vi "Get Pattern Data.vi"(9 "File Name":i32[](array[numeric]), 10 "Folder Name":string, 11 "Dispense.lvclass":refnum<class "Dispense.lvclass">) -> (3 "Dispense Out":refnum<class "Dispense.lvclass">)   [LabVIEW 2016, in "Dispense.lvclass"]
uses:
  Dispense.lvclass
  Dispense.lvclass/Dispense.ctl
panel:
  out "Timing Data (Go Down and Dispense)":T1(array[cluster])
  out "array":dbl[][](array[numeric])
  out "appended path":path
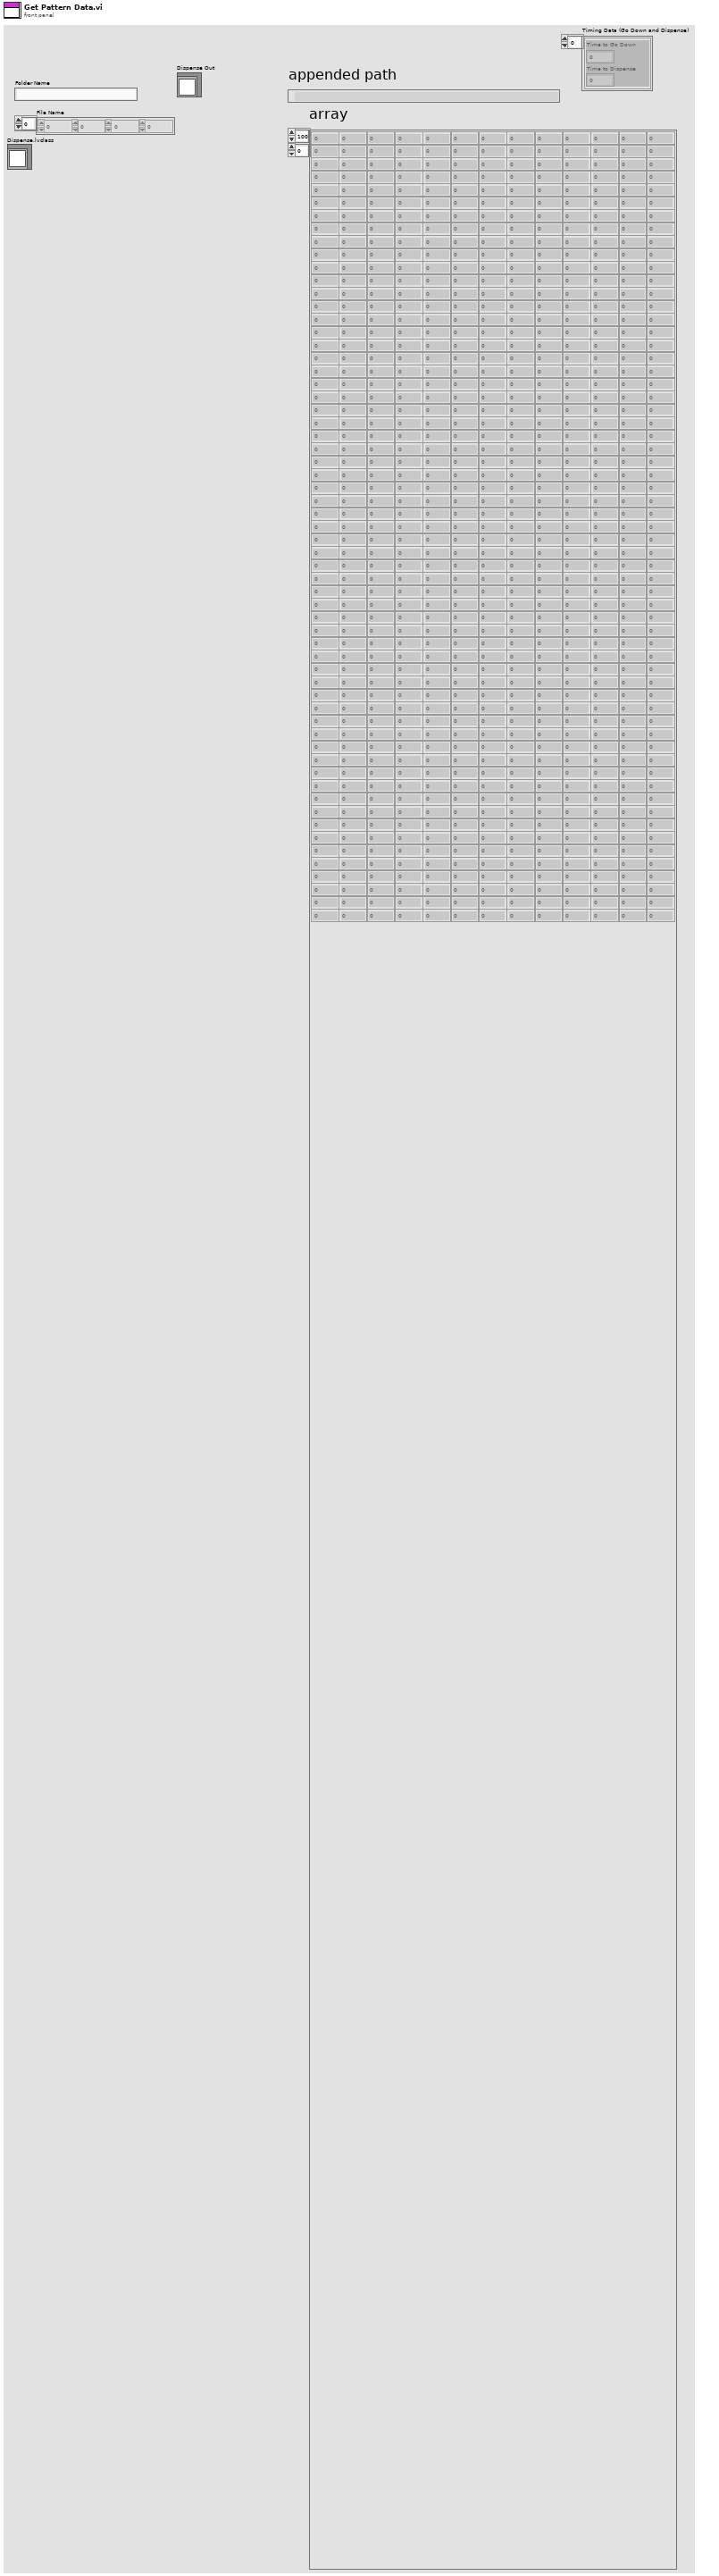
[diagram p1: front panel]
types:
  T1 = cluster{"Time to Go Down":dbl, "Time to Dispense":dbl}[]
  T2 = cluster{"Time to Go Down":dbl, "Time to Dispense":dbl}
  T3 = typedef "File Paths.ctl" = cluster{"Glue Pattern Folder":path, "Carrier Tray Folder":path, "Pick Up Tool Fixture Folder":path, "Components Folder":path, "Bellows Tool Offset.txt":path, "Pick Up Tool Offset.txt":path, "Dispense Tip Offset.txt":path, "Log Files":path}
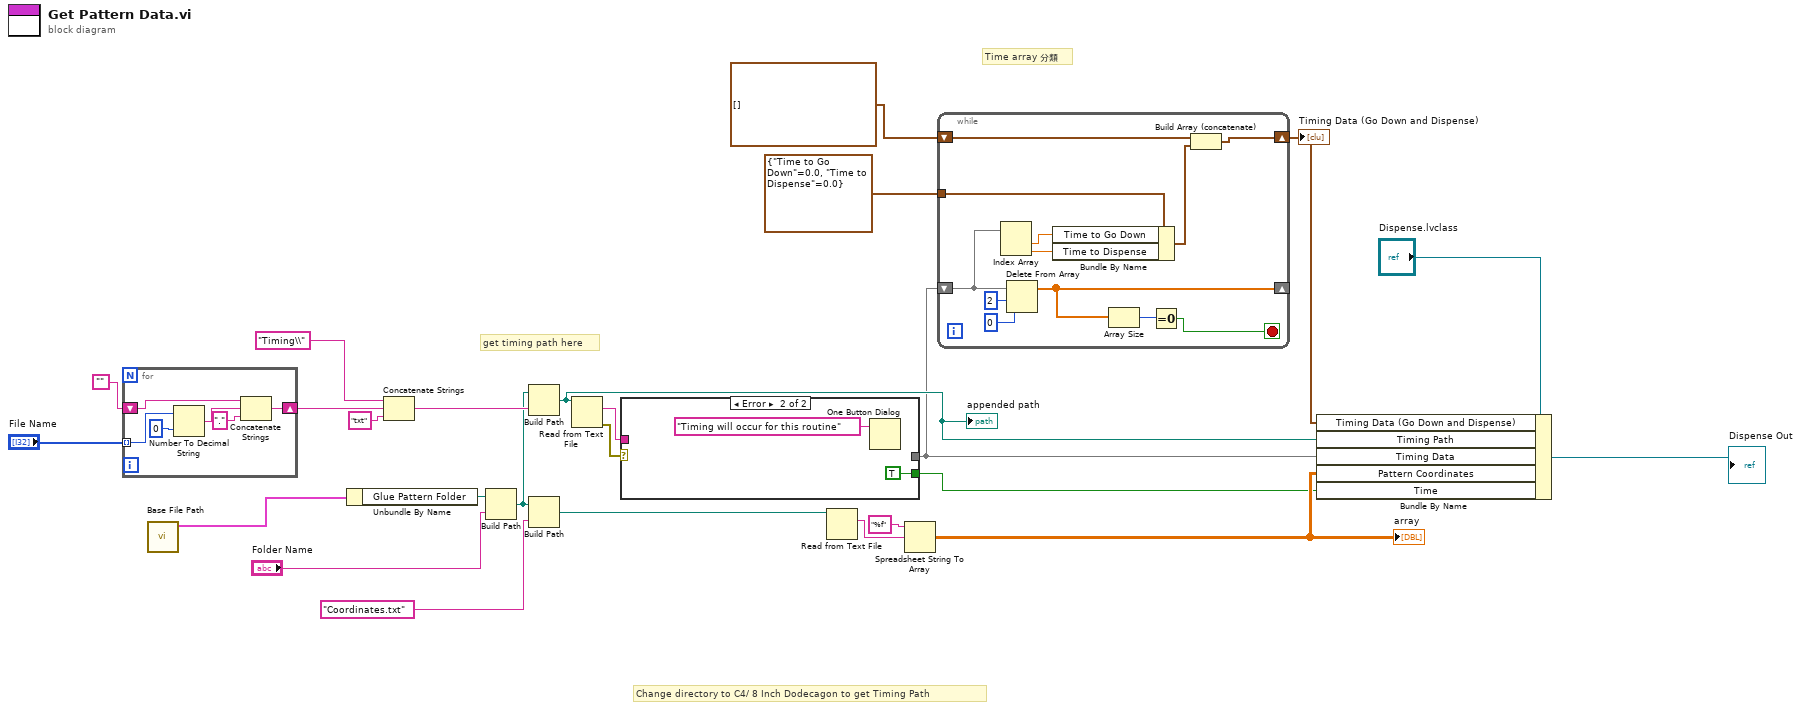
[diagram p0: block diagram]
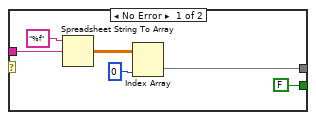
[diagram p2: hidden frame]
diagram:
  # "Time array 分類"
  # "Change directory to C4/ 8 Inch Dodecagon to get Timing Path"
  # "get timing path here"
  n1 = for {
    tunnel: "File Name" -> [w31] mode=indexing
    shift-right: [w27] -> w21
    shift-left: "" -> [w26]
    n2 = Number To Decimal String(number=w31, width (-)=i16 0) -> (decimal integer string=w29:string)
    n3 = Concatenate Strings(w26, w29, "." ("string")) -> (w27:string)
  }
  n4 = call "Base File Path.vi"() -> ("Paths Out"=w12:T3)  [unwired: 11 in]
  n5 = Unbundle By Name(w12) -> ("Glue Pattern Folder"=w16:path)
  n6 = Concatenate Strings("Timing\\" ("name or relative path"), w21, "txt" ("string")) -> (w24:string)
  n7 = Build Path(base path=w16, name or relative path="Folder Name") -> (appended path=w23:path)
  n8 = Build Path(base path=w23, name or relative path=w24) -> (appended path=w10:path)
  "appended path" <- w10
  n9 = Build Path(base path=w23, name or relative path="Coordinates.txt") -> (appended path=w18:path)
  n10 = Read from Text File(file (use dialog)=w10) -> (text=w25:string, error out=w5:errorcluster)  [unwired: 3 in, 2 out]
  n11 = case shown="Error" w5 {
    tunnel: w25 -> [w36 _]
    tunnel: [w34 _] -> w2
    tunnel: [FALSE TRUE] -> w8
    frame No Error {
      n12 = Spreadsheet String To Array(format string="%f", spreadsheet string=w36) -> (array=w35:dbl[][])  [unwired: 2 in]
      n13 = Index Array(array=w35, index (col)=0 ("disabled index (col)")) -> (element=w34:dbl[])  [unwired: 1 in]
    }
    frame Error {
      n14 = One Button Dialog(message="Timing will occur for this routine") -> ()  [unwired: 1 in, 1 out]
    }
  }
  n15 = Read from Text File(file (use dialog)=w18) -> (text=w14:string)  [unwired: 3 in, 3 out]
  n16 = Spreadsheet String To Array(format string="%f", spreadsheet string=w14) -> (array=w9:dbl[][])  [unwired: 2 in]
  "array" <- w9
  n17 = while {
    shift-right: [w50] -> w1
    shift-left: T1 [] ("Timing Data (Go Down and Dispense)") -> [w51]
    tunnel: T2 {"Time to Go Down"=0.0, "Time to Dispense"=0.0} ("Cluster") -> [w48]
    shift-right: [w40] -> _
    shift-left: w2 -> [w43]
    stop <- w44 stop-if-true
    n18 = Index Array "Index Array"(array=w43) -> (element #1=w47:dbl, element #2=w46:dbl)  [unwired: 2 in]
    n19 = Delete From Array "Delete From Array"(array=w43, length=2, index=0) -> (array with subset deleted=w40:dbl[])  [unwired: 1 out]
    n20 = Bundle By Name(cluster=w48, "Time to Go Down"=w47, "Time to Dispense"=w46) -> (w49:T2)
    n21 = Array Size(array=w40) -> (size(s)=w45:i32)
    n22 = Equal To 0?(x=w45) -> (x = 0?=w44:bool)
    n23 = Build Array (concatenate)(w51, w49) -> (w50:T1)
  }
  "Timing Data (Go Down and Dispense)" <- w1
  n24 = Bundle By Name(cluster="Dispense.lvclass", "Timing Data (Go Down and Dispense)"=w1, "Timing Path"=w10, "Timing Data"=w2, "Pattern Coordinates"=w9, "Time"=w8) -> (→"Dispense Out":refnum<class "Dispense.lvclass">)
